vi "saveparams_andscanpattern.vi"(1 "timestamp":timestamp, 2 "filename prefix in":string, 3 "data dir in":path=path "C:/Users/Labmember/Desktop/Data/temp" caption="data dir.") -> ()   [LabVIEW 2015]
panel:
  out "errors":errorcluster[](array[cluster])
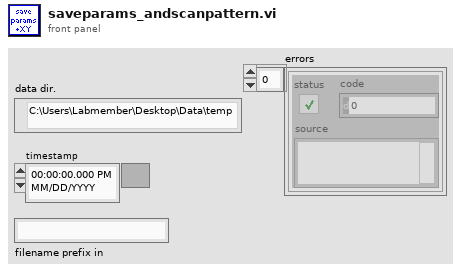
[diagram p1: front panel]
types:
  T1 = enum16{"open", "replace", "create", "open or create", "replace or create", "replace or create with confirmation"}
  T2 = enum16{"big-endian, network order", "native, host order", "little-endian"}
  T3 = typedef "LVRectTypeDef.ctl" = cluster{"Left":i16, "Top":i16, "Right":i16, "Bottom":i16}
  T4 = cluster{"Xpixels":i32, "Vxminref":dbl, "Vxmaxref":dbl, "P":dbl, "Ypixels":i32, "Vyminref":dbl, "Vymaxref":dbl, "srate":sgl, "sAOxy":i32, "timeout":dbl, "type":string, "date":string, "time":string, "Colormap":u16, "Drawing Mode":u16, "Scanning Mode":u16, "square pixels":bool, "square matrix":bool, "Xpixels Img":i32, "Vx-min Img":dbl, "VX-max Img":dbl, "Ypixels Img":i32, "Vy-min Img":dbl, "Vy-max Img ":dbl, "Angle Img":dbl, "autoshutter":bool, "finite":bool, "cont":bool, "wavdet":bool, "measpoints":i32, "avpp":i32, "bufferAO":i32, "bufferAI":i32, "starttick":u32, "waveform":path, "Vx-ref":dbl, "Vy-ref":dbl, "refreshrate":dbl, "refreshbuffer":i32, "tt_cycles":i32, "motorref":refnum<k7>, "mirrorswitch":refnum<k7>, "sample mode":i32, "maxbufferAI":i32, "srateAODO":sgl, "bin":sgl, "Pel":sgl, "Angle draw":dbl, "srate Img":sgl, "ROIimg_plotbounds":T3, "auto OD":bool, "ODfilt":u16, "aAI":i32[], "aCI":i32[], "aAO":u32[], "aDO":u32[], "refwfsize":dbl, "Lifetime":bool, "Vz-Img":dbl, "Vz-ref":dbl, "Vz-reset":dbl, "AIoverride":bool, "aAS":u32[], "XYZstart":dbl[]}
  T5 = cluster{"VC":bool, "CC":bool, "CC_icg (pA/mv)":sgl, "VC_icg (mV/mV)":sgl, "OCG (mV/pA)":sgl, "OVG (mV/mV)":dbl, "Vhold (mV)":sgl, "holdon":bool}
  T6 = cluster{"initialized":bool, "devidx":i32, "Ch0 Level":i32, "Ch0 ZeroX":i32, "Ch1 Level":i32, "Ch1 ZeroX":i32, "sync rate":i32, "resolution":i32, "acq time":i32, "acq rate":i32, "# bins":u32, "Bin size":enum16{"1", "2", "4", "8", "16", "32", "64", "128"}, "min photons":u32, "truncate":u32}
  T7 = typedef "XYZStage.lvlib/XYZStage Configuration.ctl" = cluster{"VISA resource name":refnum<visa-resource-name>, "Timeout (3sec)":u32}
  T8 = cluster{"StageS":i32, "StageL":i32, "currmeas data dir":path, "image OD":u16, "contour OD":u16, "point OD":u16, "AOlines":tag[], "AIlines":tag[], "CI lines":tag[], "DO lines":tag[], "AO names":string[], "CI names":string[], "AI names":string[], "DO names":string[], "CIextensions":string[], "AIextensions":string[], "Voltage to Ygalvo":i32, "Voltage to Xgalvo":i32, "Voltage to patch":i32, "640 shutter":i32, "2P shutter":i32, "LT timestamp":u32, "Vp":i32, "Ip":i32, "camera trigger":i32, "master data dir":path, "voltage to Zpos":i32, "Vto2P":i32, "640 AO":i32, "488 AO":i32, "532 AO":i32, "640TTL":u32, "488TTL":u32, "532TTL":u32, "Device 1 sampleclock out":tag, "Device 1 Starttrigger out":tag, "Device 2 sampleclock in":tag, "Device 2 StartTrigger in ":tag, "2PODTTL":u32, "488 shutter":u32, "LCVR red":u32, "LCVR blue":u32, "Sutter Stage Config":T7}
  T9 = cluster{"AO parameters":cluster{"AOtab":dbl, "Repeats":dbl, "Cycles":dbl, "Start amplitude (V)":dbl, "Baseline (V)":dbl, "Step size (V)":dbl, "DC (%)":dbl, "Sampling frequency (Hz)":dbl, "Period (ms)":dbl, "Offset (V)":dbl, "Amplitude (V)":dbl, "Frequency":dbl, "Tri Repeats":dbl, "phase shift (ms)":dbl, "Pulses":dbl, "Matlab wave file":path, "Tri phase":dbl, "padding value":dbl}[], "DO parameters":cluster{"Digital DC (%)":dbl, "Digital phase":dbl, "Digital Freq (Hz)":dbl, "Sampling frequency (Hz)":dbl, "Digital time offset (s) ":dbl, "padding value":dbl, "matlab wave file":path, "DOtab":dbl}[]}
  T10 = cluster{"used AO lines":tag[], "used AO names":string[]}
  T11 = cluster{"used DO lines":tag[], "used DO names":string[]}
  T12 = cluster{"params out":cluster{"Xpixels":i32, "Vxminref":dbl, "Vxmaxref":dbl, "P":dbl, "Ypixels":i32, "Vyminref":dbl, "Vymaxref":dbl, "srate":sgl, "sAOxy":i32, "timeout":dbl, "type":string, "date":string, "time":string, "Colormap":u16, "Drawing Mode":u16, "Scanning Mode":u16, "square pixels":bool, "square matrix":bool, "Xpixels Img":i32, "Vx-min Img":dbl, "VX-max Img":dbl, "Ypixels Img":i32, "Vy-min Img":dbl, "Vy-max Img ":dbl, "Angle Img":dbl, "autoshutter":bool, "finite":bool, "cont":bool, "wavdet":bool, "measpoints":i32, "avpp":i32, "bufferAO":i32, "bufferAI":i32, "starttick":u32, "waveform":path, "Vx-ref":dbl, "Vy-ref":dbl, "refreshrate":dbl, "refreshbuffer":i32, "tt_cycles":i32, "motorref":refnum<k7>, "mirrorswitch":refnum<k7>, "sample mode":i32, "maxbufferAI":i32, "srateAODO":sgl, "bin":sgl, "Pel":sgl, "Angle draw":dbl, "srate Img":sgl, "ROIimg_plotbounds":T3, "auto OD":bool, "ODfilt":u16, "aAI":i32[], "aCI":i32[], "aAO":u32[], "aDO":u32[], "refwfsize":dbl, "Lifetime":bool, "Vz-Img":dbl, "Vz-ref":dbl, "Vz-reset":dbl, "AIoverride":bool, "aAS":u32[], "XYZstart":dbl[]}, "Params out":cluster{"VC":bool, "CC":bool, "CC_icg (pA/mv)":sgl, "VC_icg (mV/mV)":sgl, "OCG (mV/pA)":sgl, "OVG (mV/mV)":dbl, "Vhold (mV)":sgl, "holdon":bool}, "Params out":cluster{"initialized":bool, "devidx":i32, "Ch0 Level":i32, "Ch0 ZeroX":i32, "Ch1 Level":i32, "Ch1 ZeroX":i32, "sync rate":i32, "resolution":i32, "acq time":i32, "acq rate":i32, "# bins":u32, "Bin size":enum16{"1", "2", "4", "8", "16", "32", "64", "128"}, "min photons":u32, "truncate":u32}, "config out":cluster{"StageS":i32, "StageL":i32, "currmeas data dir":path, "image OD":u16, "contour OD":u16, "point OD":u16, "AOlines":tag[], "AIlines":tag[], "CI lines":tag[], "DO lines":tag[], "AO names":string[], "CI names":string[], "AI names":string[], "DO names":string[], "CIextensions":string[], "AIextensions":string[], "Voltage to Ygalvo":i32, "Voltage to Xgalvo":i32, "Voltage to patch":i32, "640 shutter":i32, "2P shutter":i32, "LT timestamp":u32, "Vp":i32, "Ip":i32, "camera trigger":i32, "master data dir":path, "voltage to Zpos":i32, "Vto2P":i32, "640 AO":i32, "488 AO":i32, "532 AO":i32, "640TTL":u32, "488TTL":u32, "532TTL":u32, "Device 1 sampleclock out":tag, "Device 1 Starttrigger out":tag, "Device 2 sampleclock in":tag, "Device 2 StartTrigger in ":tag, "2PODTTL":u32, "488 shutter":u32, "LCVR red":u32, "LCVR blue":u32, "Sutter Stage Config":T7}, "Params out":cluster{"AO parameters":cluster{"AOtab":dbl, "Repeats":dbl, "Cycles":dbl, "Start amplitude (V)":dbl, "Baseline (V)":dbl, "Step size (V)":dbl, "DC (%)":dbl, "Sampling frequency (Hz)":dbl, "Period (ms)":dbl, "Offset (V)":dbl, "Amplitude (V)":dbl, "Frequency":dbl, "Tri Repeats":dbl, "phase shift (ms)":dbl, "Pulses":dbl, "Matlab wave file":path, "Tri phase":dbl, "padding value":dbl}[], "DO parameters":cluster{"Digital DC (%)":dbl, "Digital phase":dbl, "Digital Freq (Hz)":dbl, "Sampling frequency (Hz)":dbl, "Digital time offset (s) ":dbl, "padding value":dbl, "matlab wave file":path, "DOtab":dbl}[]}, cluster{"used AO lines":tag[], "used AO names":string[]}, cluster{"used DO lines":tag[], "used DO names":string[]}}
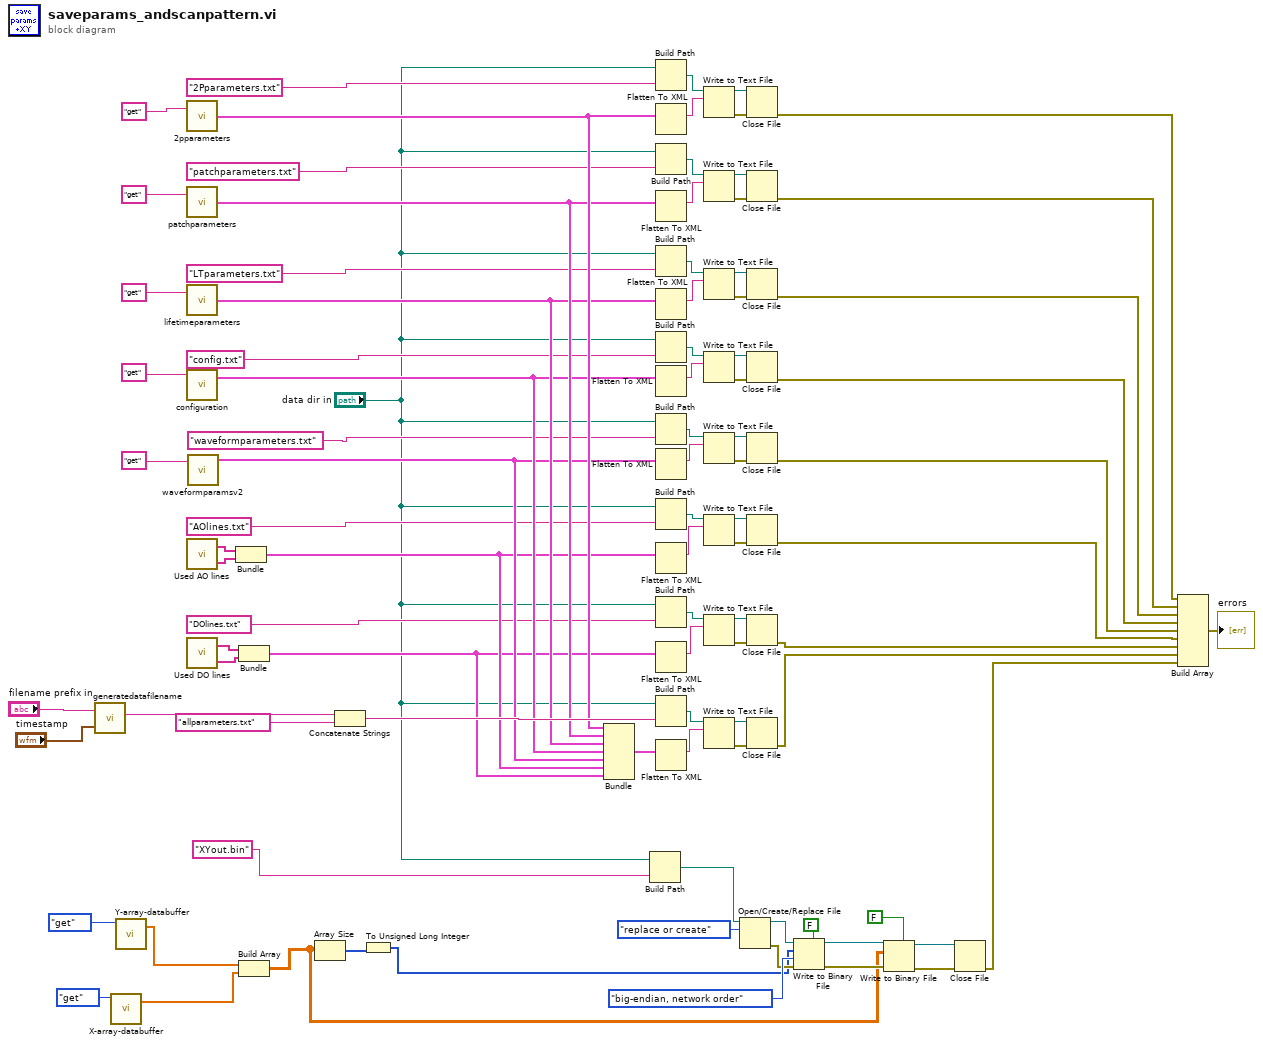
[diagram p0: block diagram]
diagram:
  n1 = call "generatedatafilename.vi"("timestamp"="timestamp", "filename prefix in"="filename prefix in") -> ("full-filename"=w44:string)
  n2 = call "X-array-databuffer.vi"("command"=enum16{"get", "set", "clear", "append"}."get") -> ("array out"=w27:dbl[])  [unwired: 3 in, 1 out]
  n3 = call "Y-array-databuffer.vi"("command"=enum16{"get", "set", "clear", "append"}."get") -> ("array out"=w28:dbl[])  [unwired: 3 in, 1 out]
  n4 = call "2pparameters.vi"("command"="get") -> ("params out"=w78:T4)  [unwired: 1 in]
  n5 = call "patchparameters.vi"("command"="get") -> ("Params out"=w73:T5)  [unwired: 1 in]
  n6 = call "lifetimeparameters.vi"("command"="get") -> ("Params out"=w68:T6)  [unwired: 1 in]
  n7 = call "configuration.vi"("command"="get") -> ("config out"=w63:T8)  [unwired: 2 in, 1 out]
  n8 = call "Used AO lines.vi"() -> ("used AO names"=w56:string[], "used AO lines"=w57:tag[])  [unwired: 2 in]
  n9 = call "Used DO lines.vi"() -> ("used DO names"=w54:string[], "used DO lines"=w55:tag[])  [unwired: 2 in]
  n10 = call "waveformparamsv2.vi"("command"="get") -> ("Params out"=w58:T9)  [unwired: 4 in, 2 out]
  n11 = Bundle("used AO lines"=w57, "used AO names"=w56) -> (w49:T10)  [unwired: 1 in]
  n12 = Bundle("used DO lines"=w55, "used DO names"=w54) -> (w43:T11)  [unwired: 1 in]
  n13 = Build Array(w28, w27) -> (w14:dbl[][])
  n14 = Array Size(array=w14) -> (size(s)=w22:i32[])
  n15 = Concatenate Strings(w44, "allparameters.txt" ("string")) -> (w90:string)
  n16 = To Unsigned Long Integer(number=w22) -> (unsigned 32bit integer=w21:u32[])
  n17 = Bundle("params out"=w78, "Params out"=w73, "Params out"=w68, "config out"=w63, "Params out"=w58, w49, w43) -> (w86:T12)  [unwired: 1 in]
  n18 = Build Path(base path="data dir in", name or relative path="XYout.bin" ("string")) -> (appended path=w18:path)
  n19 = Build Path(base path="data dir in", name or relative path="2Pparameters.txt" ("string")) -> (appended path=w79:path)
  n20 = Flatten To XML(anything=w78) -> (xml string=w82:string)
  n21 = Build Path(base path="data dir in", name or relative path="patchparameters.txt" ("string")) -> (appended path=w77:path)
  n22 = Flatten To XML(anything=w73) -> (xml string=w74:string)
  n23 = Build Path(base path="data dir in", name or relative path="LTparameters.txt" ("string")) -> (appended path=w69:path)
  n24 = Flatten To XML(anything=w68) -> (xml string=w72:string)
  n25 = Build Path(base path="data dir in", name or relative path="config.txt" ("string")) -> (appended path=w67:path)
  n26 = Flatten To XML(anything=w63) -> (xml string=w64:string)
  n27 = Build Path(base path="data dir in", name or relative path="waveformparameters.txt" ("string")) -> (appended path=w59:path)
  n28 = Flatten To XML(anything=w58) -> (xml string=w62:string)
  n29 = Build Path(base path="data dir in", name or relative path="AOlines.txt" ("string")) -> (appended path=w53:path)
  n30 = Flatten To XML(anything=w49) -> (xml string=w50:string)
  n31 = Build Path(base path="data dir in", name or relative path="DOlines.txt" ("string")) -> (appended path=w45:path)
  n32 = Flatten To XML(anything=w43) -> (xml string=w48:string)
  n33 = Build Path(base path="data dir in", name or relative path=w90) -> (appended path=w87:path)
  n34 = Flatten To XML(anything=w86) -> (xml string=w85:string)
  n35 = Write to Text File(file (use dialog)=w79, text=w82) -> (refnum out=w80:refnum<file>, error out=w81:errorcluster)  [unwired: 2 in, 1 out]
  n36 = Write to Text File(file (use dialog)=w77, text=w74) -> (refnum out=w76:refnum<file>, error out=w75:errorcluster)  [unwired: 2 in, 1 out]
  n37 = Write to Text File(file (use dialog)=w69, text=w72) -> (refnum out=w70:refnum<file>, error out=w71:errorcluster)  [unwired: 2 in, 1 out]
  n38 = Write to Text File(file (use dialog)=w67, text=w64) -> (refnum out=w66:refnum<file>, error out=w65:errorcluster)  [unwired: 2 in, 1 out]
  n39 = Write to Text File(file (use dialog)=w59, text=w62) -> (refnum out=w60:refnum<file>, error out=w61:errorcluster)  [unwired: 2 in, 1 out]
  n40 = Write to Text File(file (use dialog)=w53, text=w50) -> (refnum out=w52:refnum<file>, error out=w51:errorcluster)  [unwired: 2 in, 1 out]
  n41 = Write to Text File(file (use dialog)=w45, text=w48) -> (refnum out=w46:refnum<file>, error out=w47:errorcluster)  [unwired: 2 in, 1 out]
  n42 = Write to Text File(file (use dialog)=w87, text=w85) -> (refnum out=w89:refnum<file>, error out=w88:errorcluster)  [unwired: 2 in, 1 out]
  n43 = Open/Create/Replace File(file path (use dialog)=w18, operation (0:open)=T1."replace or create") -> (refnum out=w24:refnum<file>, error out=w23:errorcluster)  [unwired: 4 in, 1 out]
  n44 = Close File(refnum=w80, error in=w81) -> (error out=w10:errorcluster)  [unwired: 1 out]
  n45 = Close File(refnum=w76, error in=w75) -> (error out=w9:errorcluster)  [unwired: 1 out]
  n46 = Close File(refnum=w70, error in=w71) -> (error out=w8:errorcluster)  [unwired: 1 out]
  n47 = Close File(refnum=w66, error in=w65) -> (error out=w7:errorcluster)  [unwired: 1 out]
  n48 = Close File(refnum=w60, error in=w61) -> (error out=w6:errorcluster)  [unwired: 1 out]
  n49 = Close File(refnum=w52, error in=w51) -> (error out=w5:errorcluster)  [unwired: 1 out]
  n50 = Close File(refnum=w46, error in=w47) -> (error out=w4:errorcluster)  [unwired: 1 out]
  n51 = Close File(refnum=w89, error in=w88) -> (error out=w3:errorcluster)  [unwired: 1 out]
  n52 = Write to Binary File(file (use dialog)=w24, data=w21, error in=w23, 5:FALSE ("prepend array or string size? (T)"), 9:T2."big-endian, network order" ("byte order (0:big-endian, network order)")) -> (refnum out=w16:refnum<file>, error out=w15:errorcluster)  [unwired: 1 in, 1 out]
  n53 = Write to Binary File(file (use dialog)=w16, data=w14, error in=w15, 5:FALSE ("prepend array or string size? (T)")) -> (refnum out=w13:refnum<file>, error out=w12:errorcluster)  [unwired: 2 in, 1 out]
  n54 = Close File(refnum=w13, error in=w12) -> (error out=w2:errorcluster)  [unwired: 1 out]
  n55 = Build Array(w10, w9, w8, w7, w6, w5, w4, w3, w2) -> (→"errors":errorcluster[])
